vi "Reset Meas v 4.vi"(11 "simulate":bool) -> (0 "Reset Error":bool)   [LabVIEW 2013]
uses:
  <vilib>/Platform/TimedLoop/XDataNode/timing_clust.ctl
  <vilib>/Platform/TimedLoop/XDataNode/nitl_modes.ctl
  <vilib>/Platform/TimedLoop/XDataNode/wakeup.ctl
  <vilib>/platform/TimedLoop/XDataNode/XDataNode.xnode
  <vilib>/Platform/TimedLoop/XDataNode/XDNodeRunTimeDep.lvlib
panel:
  out "Reset Time Out":dbl
  out "A-D Loop Time":dbl
  out "Message":string
  in  "End Reset Routine":bool
  # "USB RESET BUSY"
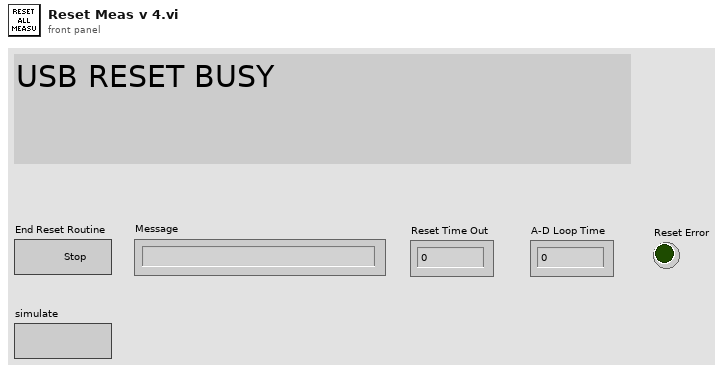
[diagram p1: front panel]
types:
  T1 = typedef "XDNodeRunTimeDep.lvlib/timing_clust.ctl" = cluster{"Expected End [f-1]":u64, "Actual End [f-1]":u64, "Finished Late? [f-1]":bool, "Expected End [i-1]":u64, "Actual End [i-1]":u64, "Finished Late? [i-1]":bool, "Expected Start [i]":u64, "Actual Start [i]":u64, "Expected Start [f]":u64, "Actual Start [f]":u64, "Source Name":string, "Structure Name":string, "Period":i64, "Deadline":i64, "Offset":i64, "Start":i64, "Priority":i32, "Timeout":i32, "Mode":T2, "Wakeup Reason":T3, "Error":errorcluster, "Source Type":string, "Secondary Source Type":string, "Global End Time":u64, "Global Start Time":u64, "Frame Duration":u64, "Iteration Duration":u64, "Assigned CPU":i32, "I/O Scan Engine Mode":u32}
  T2 = typedef "XDNodeRunTimeDep.lvlib/nitl_modes.ctl" = enum32{"No Change", "Process missed periods, maintain original phase", "Discard missed periods, maintain original phase", "Process missed periods, ignore original phase", "Discard missed periods, ignore original phase"}
  T3 = typedef "XDNodeRunTimeDep.lvlib/wakeup.ctl" = enum32{"Normal", "Aborted", "Asynchronous wakeup", "Timing source error", "Timed loop error", "Timeout"}
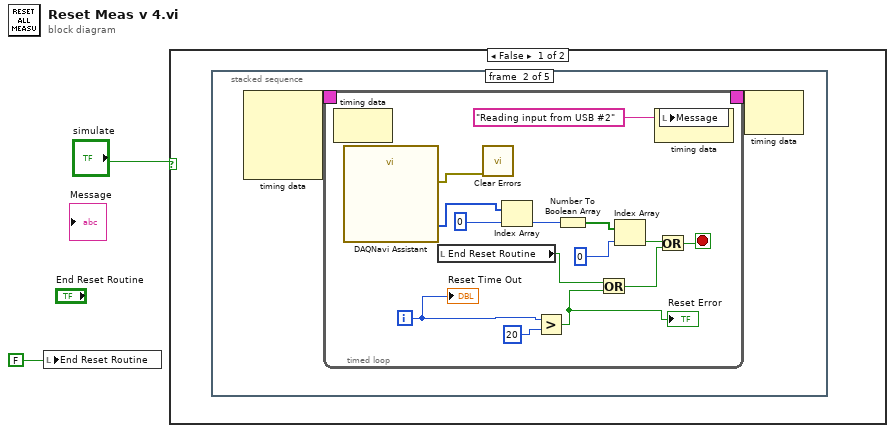
[diagram p0: block diagram]
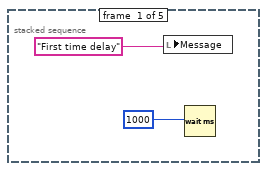
[diagram p2: hidden frame]
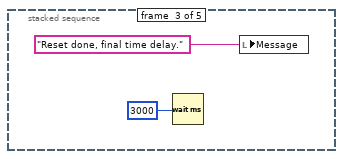
[diagram p3: hidden frame]
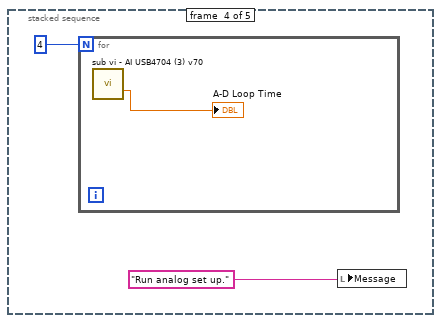
[diagram p4: hidden frame]
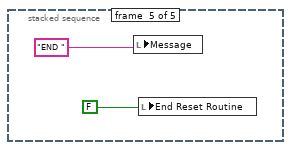
[diagram p5: hidden frame]
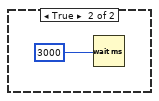
[diagram p6: hidden frame]
diagram:
  n1 = local write "End Reset Routine"(FALSE) -> ()
  n2 = case shown="False" "simulate" {
    frame False {
      n3 = stacked-sequence {
        frame #0 {
          n4 = local write "Message"("First time delay") -> ()
          n5 = Wait (ms)(milliseconds to wait=1000) -> ()  [unwired: 1 out]
        }
        frame #1 {
          n6 = node-c288() -> (w6:T1)  [unwired: 4 in]
          n7 = timed-loop {
            timing: w6 -> [_]
            timing-out: [_] -> w5
            i -> [w7]
            stop <- w16 stop-if-true
            n8 = node-c288() -> ()  [unwired: 1 in, 1 out]
            n9 = call "DAQNavi Assistant"() -> ("error out"=w12:errorcluster, "dataOut(U8Array)"=w13:u8[])  [unwired: 26 in]
            n10 = local read "End Reset Routine"() -> (w11:bool)
            n11 = call <vilib>:"Clear Errors.vi"("error in (no error)"=w12) -> ()  [unwired: 6 in, 1 out]
            n12 = Index Array(array=w13, index=0) -> (element=w18:u8)
            n13 = Greater?(x=w7, y=20) -> (0:w8:bool)
            "Reset Error" <- w8
            n14 = Number To Boolean Array(number=w18) -> (Boolean array=w19:bool[])
            n15 = Or(x=w11, y=w8) -> (x .or. y?=w9:bool)
            n16 = Index Array(array=w19, index=0) -> (element=w15:bool)
            n17 = node-c288() -> ()  [unwired: 1 in, 1 out]
            n18 = Or(x=w15, y=w9) -> (x .or. y?=w16:bool)
            n19 = local write "Message"("Reading input from USB #2") -> ()
            "Reset Time Out" <- w7
          }
          n20 = node-c288(w5) -> ()  [unwired: 1 out]
        }
        frame #2 {
          n21 = Wait (ms)(milliseconds to wait=3000) -> ()  [unwired: 1 out]
          n22 = local write "Message"("Reset done, final time delay.") -> ()
        }
        frame #3 {
          n23 = for {
            N: 4 -> [_]
            n24 = call "sub vi - AI USB4704 (3) v70.vi"() -> ("loop time"=→"A-D Loop Time":dbl)  [unwired: 11 in, 4 out]
          }
          n25 = local write "Message"("Run analog set up.") -> ()
        }
        frame #4 {
          n26 = local write "Message"("END ") -> ()
          n27 = local write "End Reset Routine"(FALSE) -> ()
        }
      }
    }
    frame True {
      n28 = Wait (ms)(milliseconds to wait=3000) -> ()  [unwired: 1 out]
    }
  }
